vi "IFD Image Write to File.vi"(8 "error in (no error)":errorcluster, 10 "refnum in":refnum<file>, 11 "IFD in":refnum<class "IFD.lvclass">) -> (0 "error out":errorcluster, 2 "refnum out":refnum<file>)   [LabVIEW 2016, in "IFD.lvclass"]
uses:
  IFD.lvclass
  IFD.lvclass/IFD.ctl
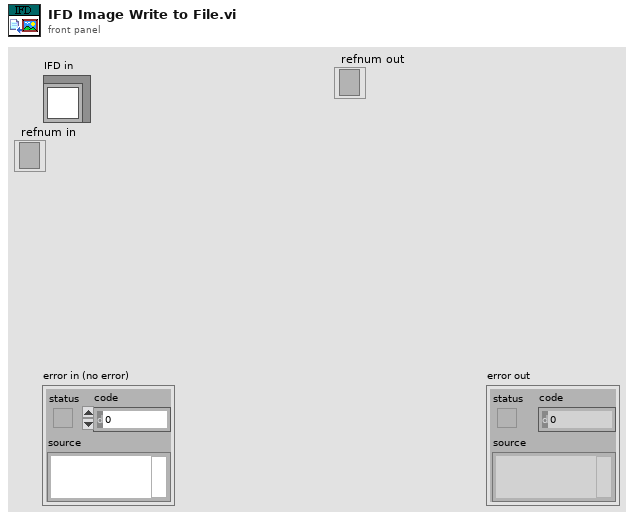
[diagram p1: front panel]
types:
  T1 = typedef "Img Data Type.ctl" = enum16{"U16", "RGB", "SGL"}
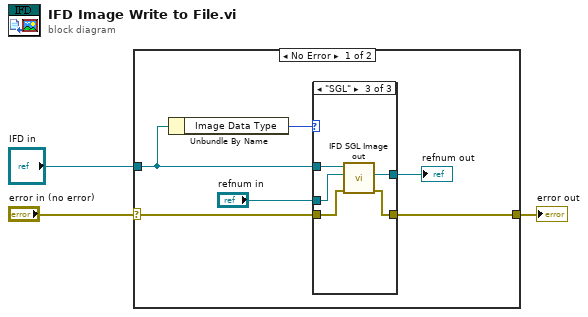
[diagram p0: block diagram]
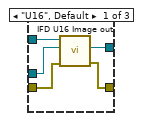
[diagram p2: hidden frame]
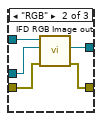
[diagram p3: hidden frame]
diagram:
  n1 = case shown="No Error" "error in (no error)" {
    selector: "error in (no error)" -> [w6 w25]
    tunnel: [w4 w25] -> w2
    tunnel: "IFD in" -> [w8 _]
    frame No Error {
      n2 = Unbundle By Name(w8) -> ("Image Data Type"=w9:T1)
      n3 = case shown="\"SGL\"" w9 {
        tunnel: w8 -> [w14 w19 w24]
        tunnel: "refnum in" -> [w13 w18 w23]
        tunnel: w6 -> [w11 w17 w22]
        tunnel: [w12 w16 w21] -> w5
        tunnel: [w10 w15 w20] -> w4
        frame "U16", Default {
          n4 = call "IFD U16 Image out.vi"("error in (no error)"=w11, "refnum in"=w13, "IFD in"=w14) -> ("error out"=w10:errorcluster, "refnum out"=w12:refnum<file>)  [unwired: 7 in]
        }
        frame "RGB" {
          n5 = call "IFD RGB Image out.vi"("error in (no error)"=w17, "refnum in"=w18, "IFD in"=w19) -> ("error out"=w15:errorcluster, "refnum out"=w16:refnum<file>)  [unwired: 7 in]
        }
        frame "SGL" {
          n6 = call "IFD SGL Image out.vi"("error in (no error)"=w22, "refnum in"=w23, "IFD in"=w24) -> ("error out"=w20:errorcluster, "refnum out"=w21:refnum<file>)  [unwired: 7 in]
        }
      }
      "refnum out" <- w5
    }
    frame Error {
    }
  }
  "error out" <- w2
